vi "Destroy EUI Events.vi"(8 "error in (no error)":errorcluster, 11 "EUI Events in":refnum<class "EUI Events.lvclass">) -> (0 "error out":errorcluster, 3 "EUI Events out":refnum<class "EUI Events.lvclass">)   [LabVIEW 2016, in "EUI Events.lvclass"]
uses:
  EUI Events.lvclass
  EUI Events.lvclass/EUI Events.ctl
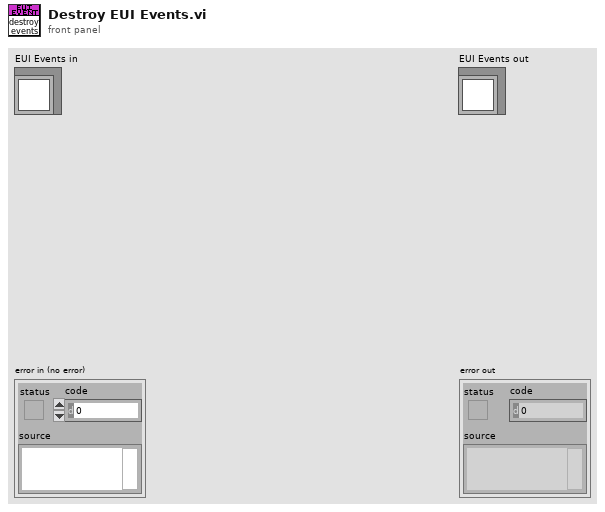
[diagram p1: front panel]
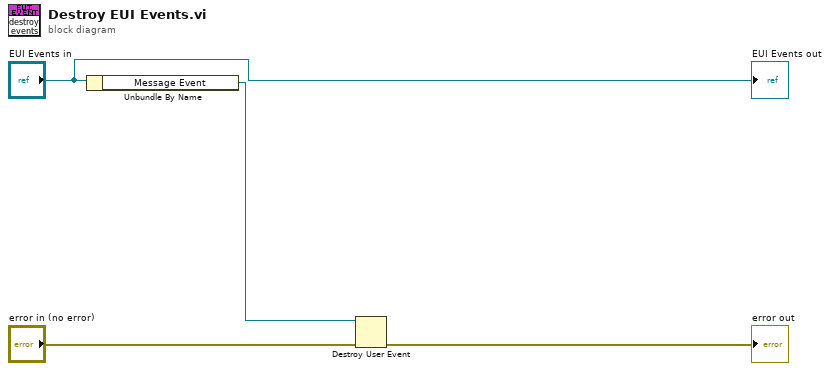
[diagram p0: block diagram]
diagram:
  n1 = Unbundle By Name("EUI Events in") -> ("Message Event"=w4:refnum<user-event>)
  n2 = Destroy User Event(user event=w4, error in="error in (no error)") -> (error out=→"error out":errorcluster)
  "EUI Events out" <- "EUI Events in"
